vi "Main HMI.vi"() -> ()   [LabVIEW 2020]
uses:
  Control/State - Main HMI.ctl
  Control/Button Strip.ctl
  Control/State - eFGV.ctl
panel:
  in  "EXIT Button":bool
  out "error out":errorcluster
  in  "error in (no error)":errorcluster
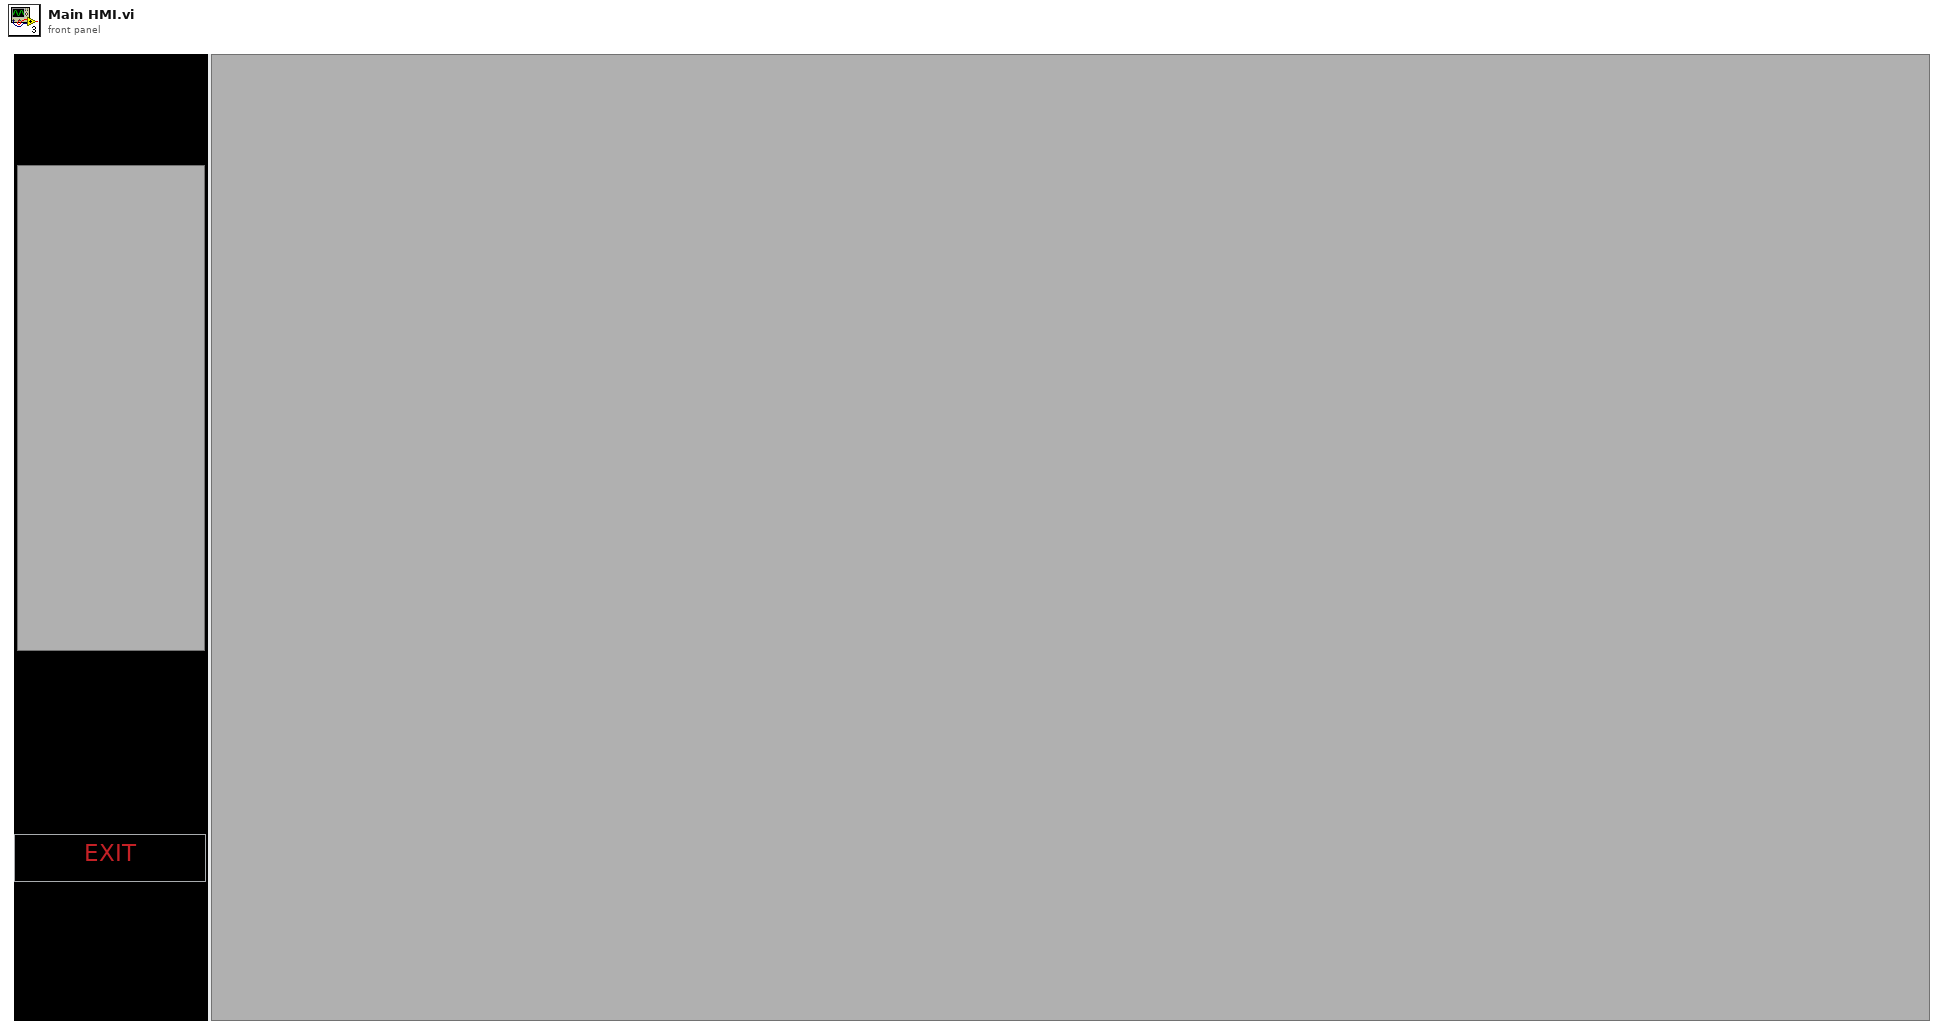
[diagram p1: front panel]
types:
  T1 = typedef "Button Strip.ctl" = enum32{"Home", "Setting", "Alert", "Save", "Chart"}
  T2 = cluster{"Timeout":i32, "Radio Buttons":T1, "All Module Ref":refnum<vi>[]}
  T3 = typedef "State - Main HMI.ctl" = enum16{"Init module", "Register event", "Init eFGV", "Run Module", "Idle", "Change Page", "Request Data from Modbus", "Process Data", "Update Layout", "Send to SQL Module", "Close All Module", "Unregister event", "Close module"}
  T4 = typedef "State - eFGV.ctl" = enum16{"Init", "Read", "Write", "Close"}
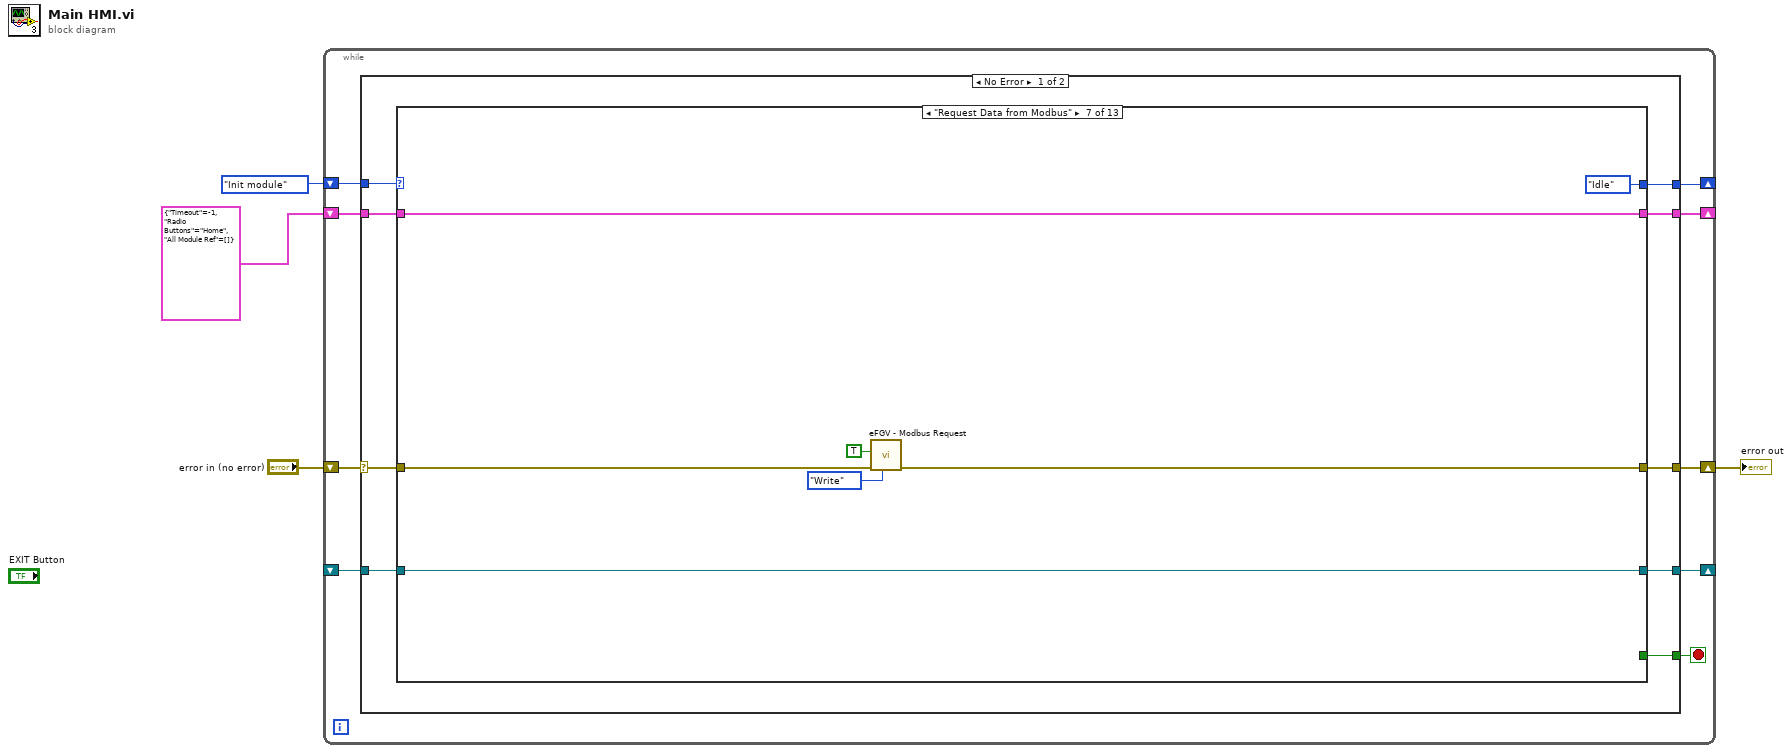
[diagram p0: block diagram]
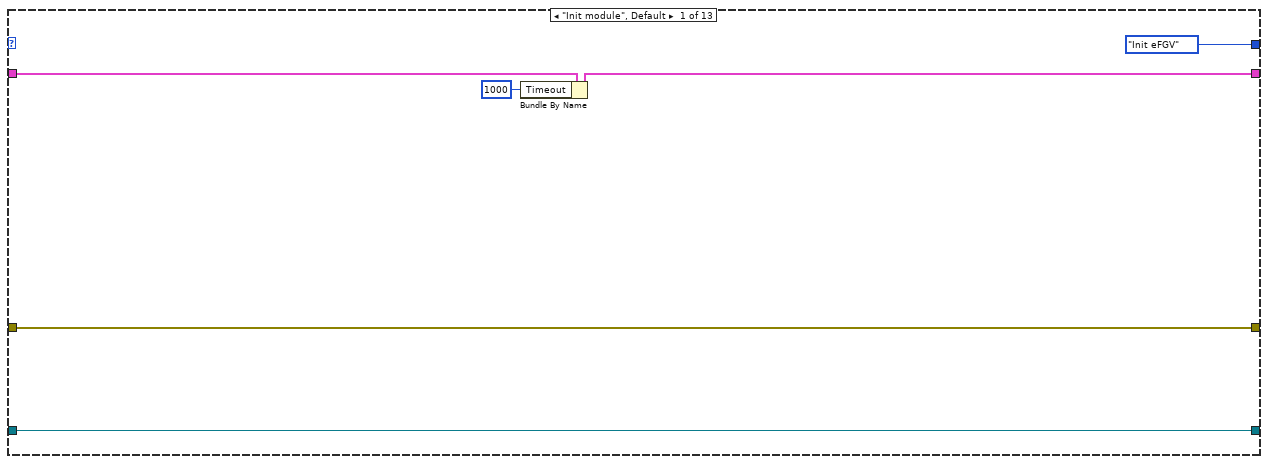
[diagram p2: hidden frame]
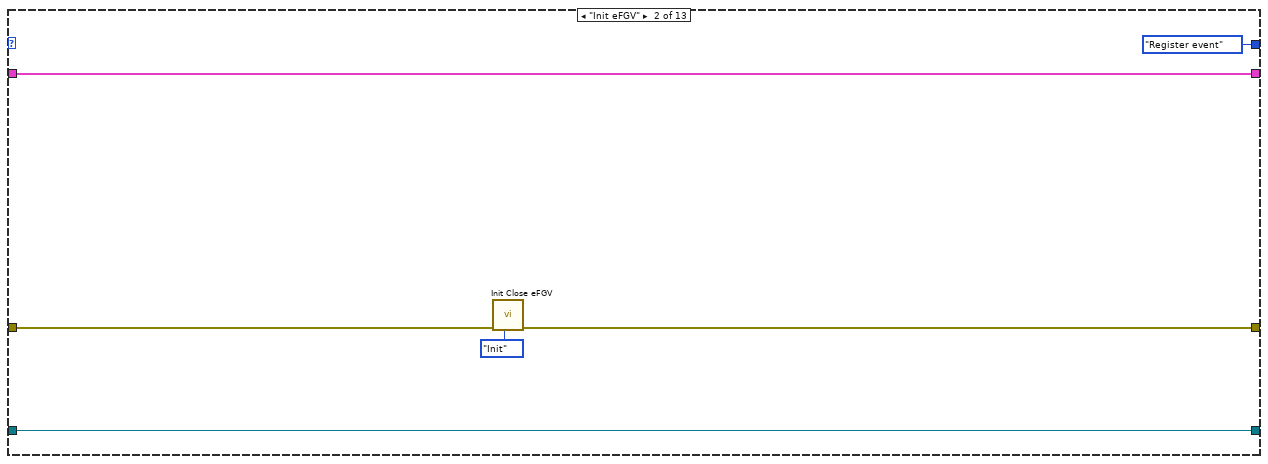
[diagram p3: hidden frame]
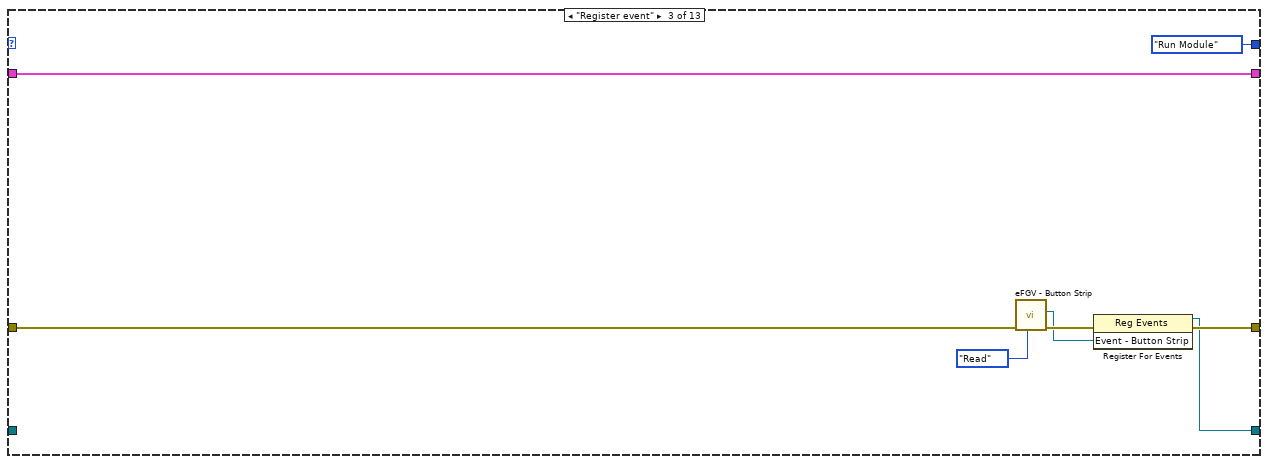
[diagram p4: hidden frame]
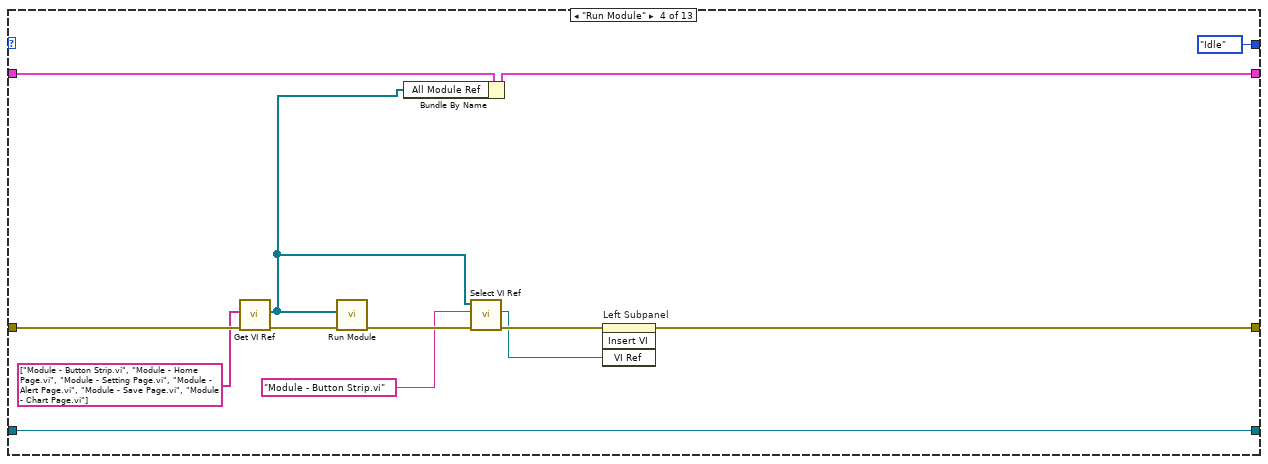
[diagram p5: hidden frame]
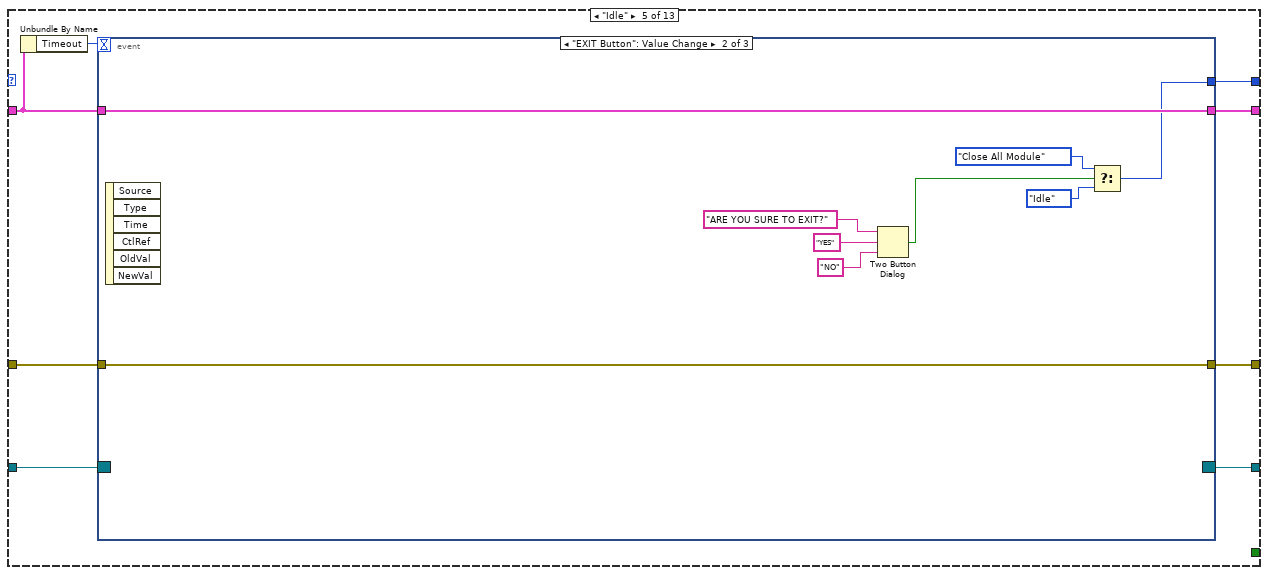
[diagram p6: hidden frame]
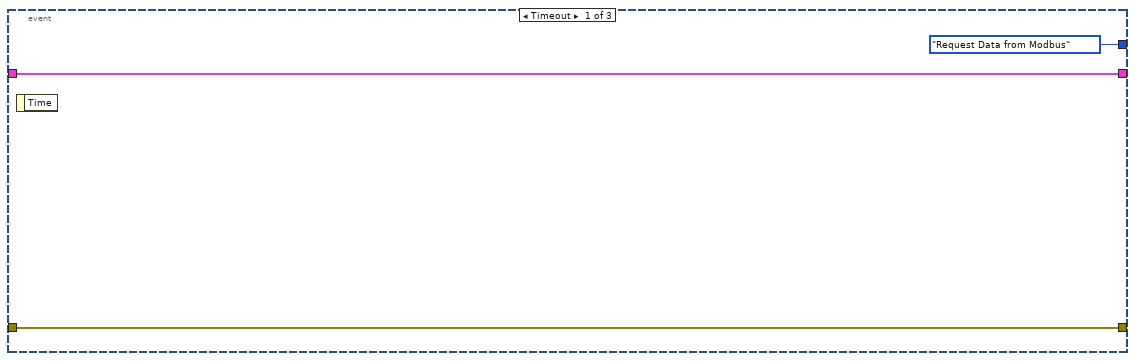
[diagram p7: hidden frame]
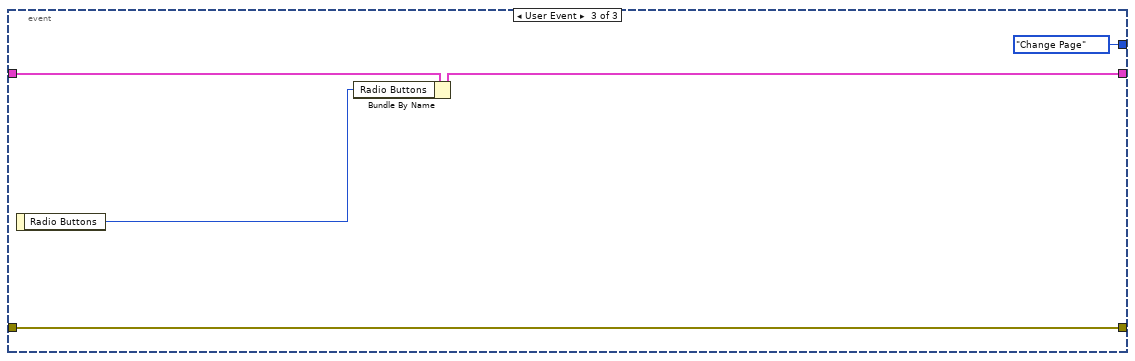
[diagram p8: hidden frame]
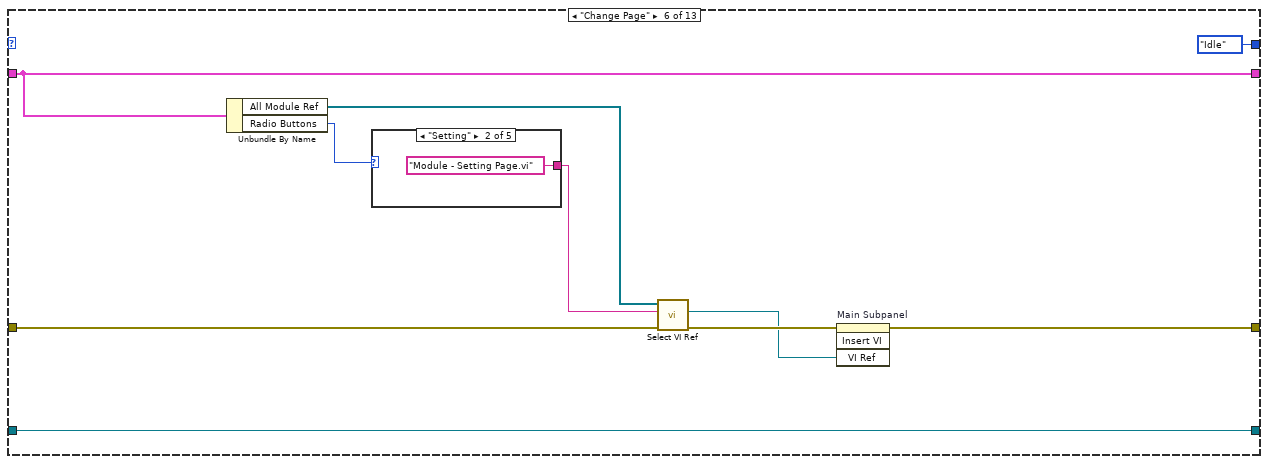
[diagram p9: hidden frame]
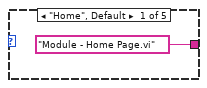
[diagram p10: hidden frame]
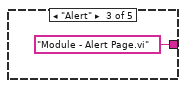
[diagram p11: hidden frame]
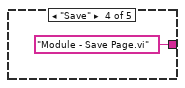
[diagram p12: hidden frame]
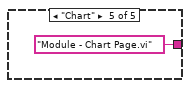
[diagram p13: hidden frame]
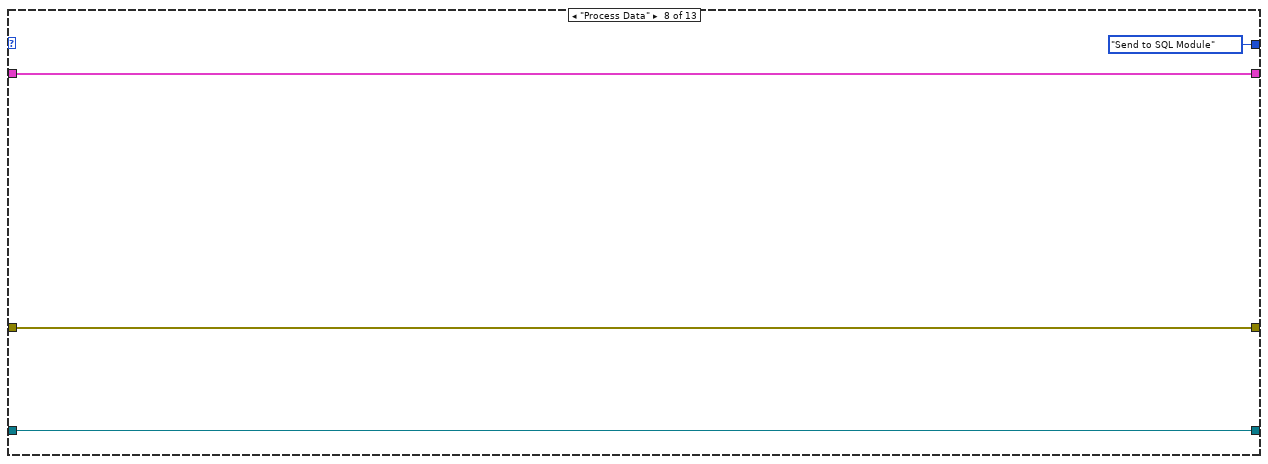
[diagram p14: hidden frame]
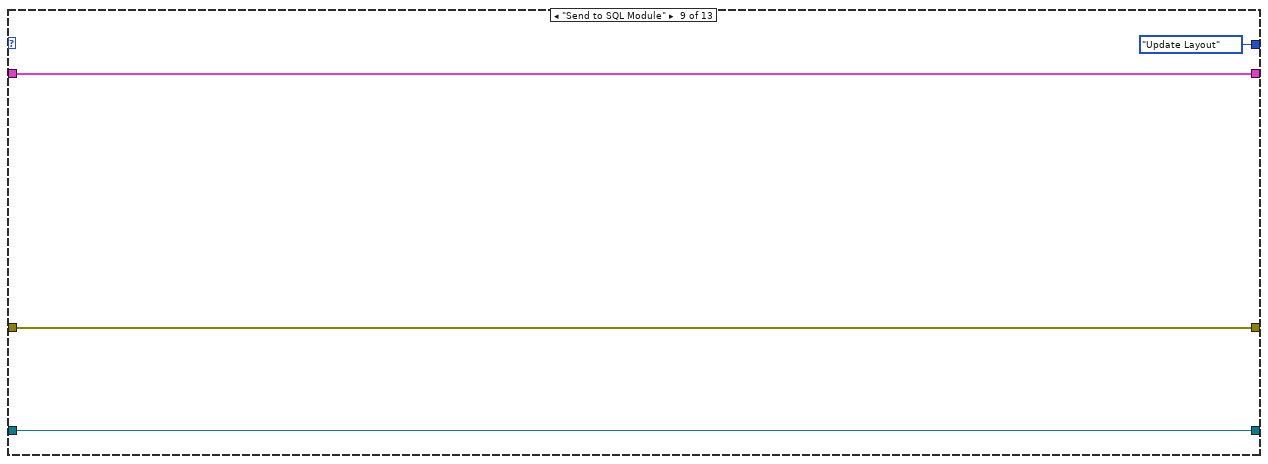
[diagram p15: hidden frame]
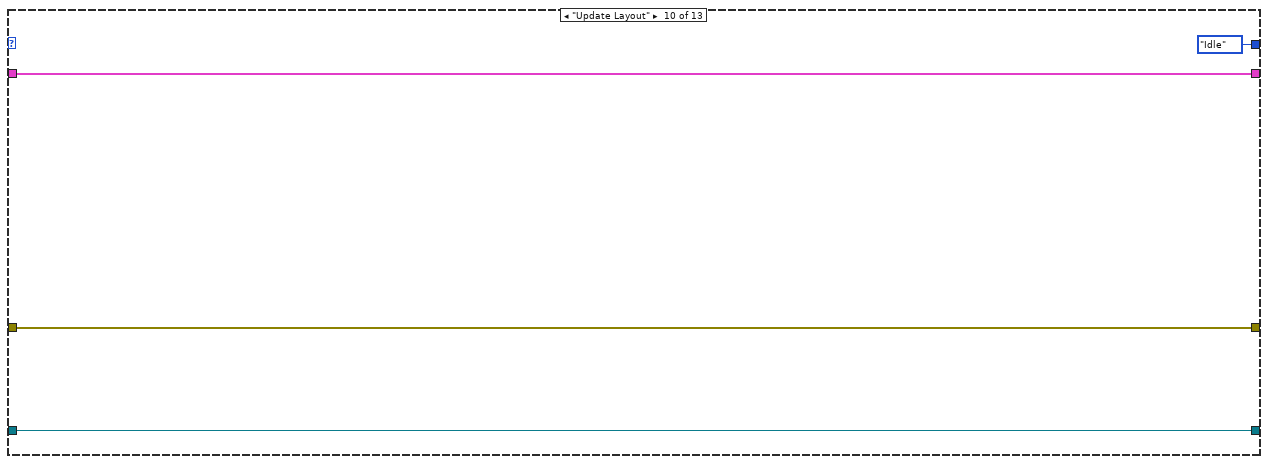
[diagram p16: hidden frame]
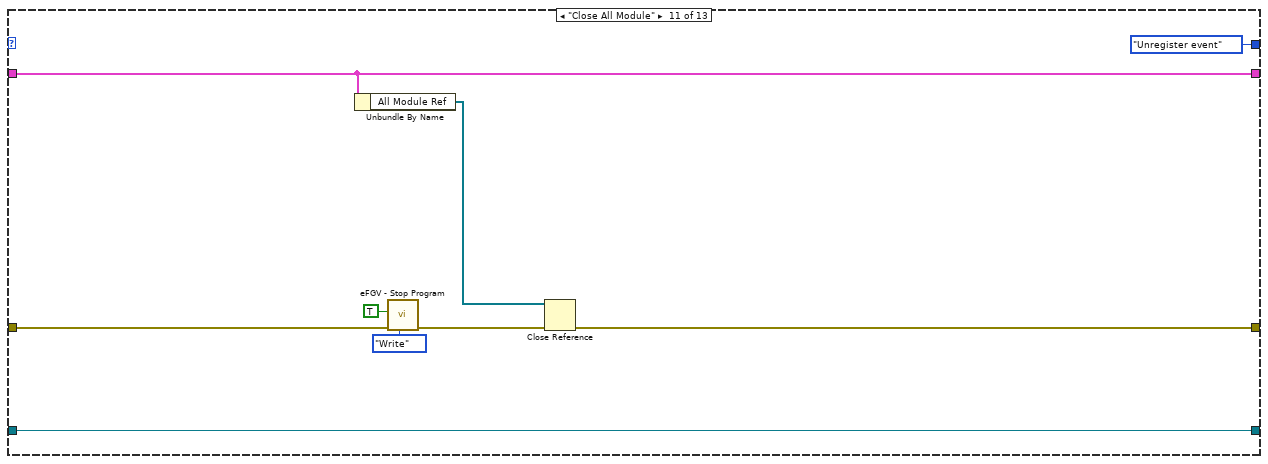
[diagram p17: hidden frame]
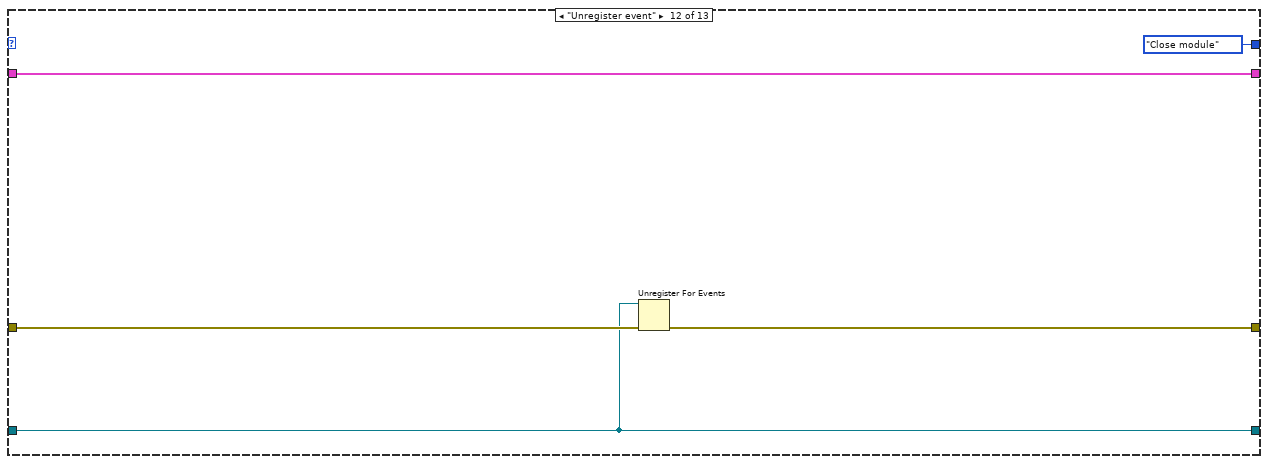
[diagram p18: hidden frame]
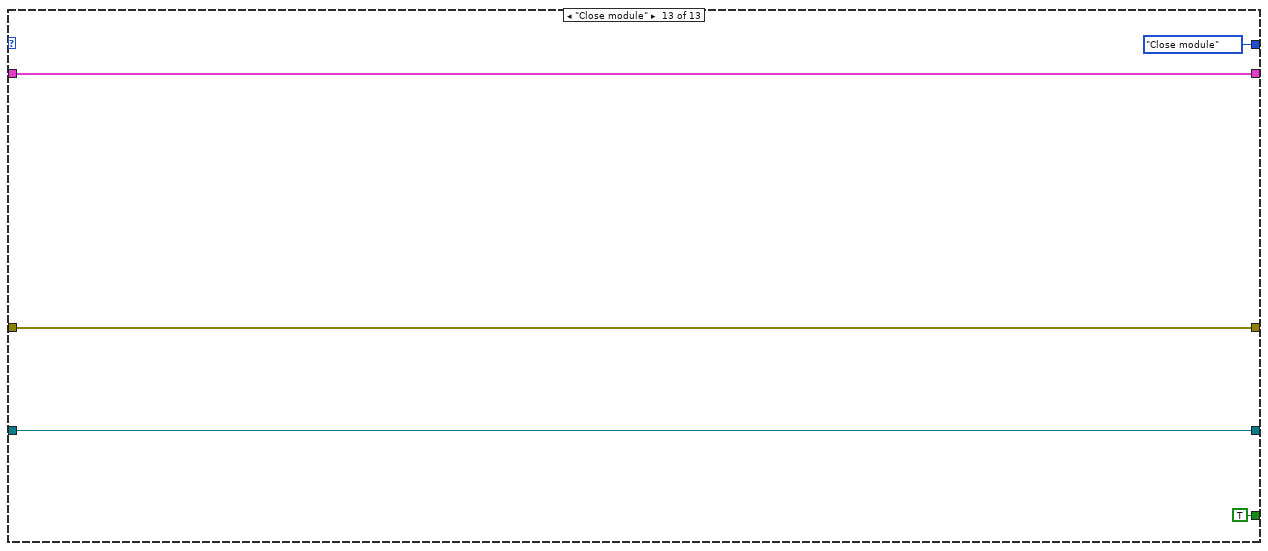
[diagram p19: hidden frame]
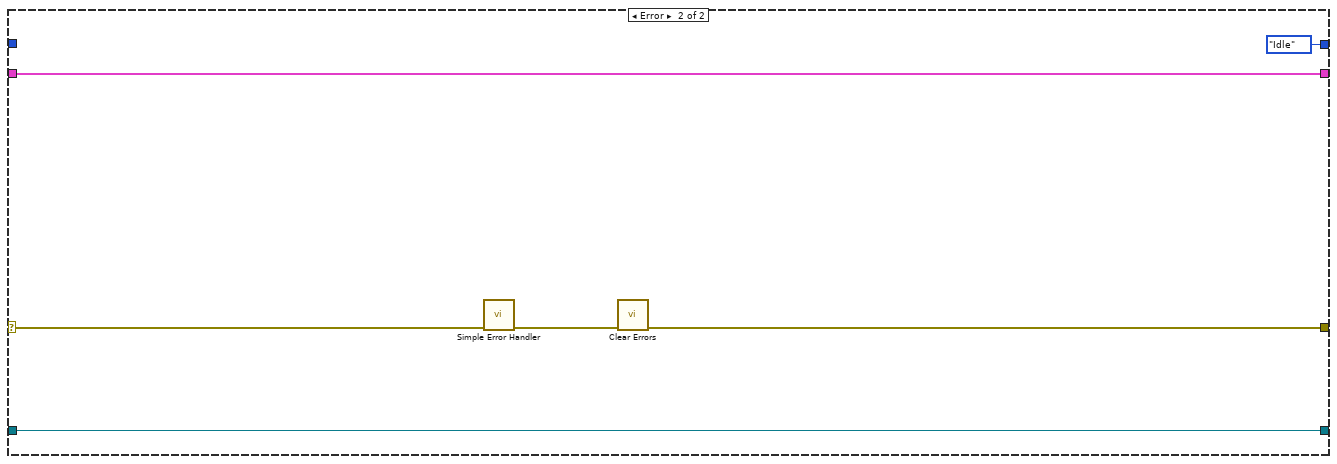
[diagram p20: hidden frame]
diagram:
  n1 = while {
    shift-right: [w11] -> w3
    shift-left: "error in (no error)" -> [w13]
    shift-right: [w7] -> _
    shift-left: State_-_Main_HMI."Init module" -> [w12]
    shift-right: [w9] -> _
    shift-left: T2 {"Timeout"=-1, "Radio Buttons"=enum."Home", "All Module Ref"=[]} -> [w10]
    shift-right: [w6] -> _
    shift-left: _ -> [w5]
    stop <- w8 stop-if-true
    n2 = case shown="No Error" w13 {
      selector: w13 -> [w21 w139]
      tunnel: w12 -> [w22 _]
      tunnel: [w20 w135] -> w11
      tunnel: w10 -> [w19 w137]
      tunnel: [w18 w137] -> w9
      tunnel: [w17 _] -> w8
      tunnel: [w16 State_-_Main_HMI."Idle"] -> w7
      tunnel: [w15 w134] -> w6
      tunnel: w5 -> [w14 w134]
      frame No Error {
        n3 = case shown="\"Request Data from Modbus\"" w22 {
          tunnel: w21 -> [w28 w31 w37 w54 w60 w87 w99 w106 w110 w114 w122 w127 w133]
          tunnel: [w28 w30 w40 w44 w59 w90 w98 w106 w110 w114 w116 w126 w133] -> w20
          tunnel: w19 -> [w27 w34 w42 w51 w62 w84 w102 w105 w109 w113 w118 w128 w132]
          tunnel: [w25 w34 w42 w50 w61 w84 w102 w105 w109 w113 w118 w128 w132] -> w18
          tunnel: [_ _ _ _ _ _ _ _ _ _ _ _ TRUE] -> w17
          tunnel: [State_-_Main_HMI."Init eFGV" State_-_Main_HMI."Register event" State_-_Main_HMI."Run Module" State_-_Main_HMI."Idle" w58 State_-_Main_HMI."Idle" State_-_Main_HMI."Idle" State_-_Main_HMI."Send to SQL Module" State_-_Main_HMI."Update Layout" State_-_Main_HMI."Idle" State_-_Main_HMI."Unregister event" State_-_Main_HMI."Close module" State_-_Main_HMI."Close module"] -> w16
          tunnel: [w23 w32 w39 w52 w56 w89 w100 w103 w107 w111 w119 w124 w129] -> w15
          tunnel: w14 -> [w23 w32 _ w52 w57 w89 w100 w103 w107 w111 w119 w124 w129]
          frame "Init module", Default {
            n4 = Bundle By Name(cluster=w27, "Timeout"=1000) -> (w25:T2)
          }
          frame "Init eFGV" {
            n5 = call "Init Close eFGV.vi"("State - eFGV"=State_-_eFGV."Init", "error in (no error)"=w31) -> ("error out"=w30:errorcluster)  [unwired: 9 in]
          }
          frame "Register event" {
            n6 = call "eFGV - Button Strip.vi"("State - eFGV"=State_-_eFGV."Read", "error in (no error)"=w37) -> ("error out"=w38:errorcluster, "Event - Button Strip"=w36:refnum<user-event>)  [unwired: 8 in]
            n7 = register-events(error in=w38, w36) -> (reference out=w39:refnum<event-registration>, error out=w40:errorcluster)  [unwired: 1 in]
          }
          frame "Run Module" {
            n8 = call "Get VI Ref.vi"("error in (no error)"=w54, "Module Names"=string[] ["Module - Button Strip.vi", "Module - Home Page.vi", "Module - Setting Page.vi", "Module - Alert Page.vi", "Module - Save Page.vi", "Module - Chart Page.vi"]) -> ("error out"=w49:errorcluster, "All Module Ref"=w47:refnum<vi>[])  [unwired: 8 in]
            n9 = call "Run Module.vi"("error in (no error)"=w49, "All Module Ref"=w47) -> ("error out"=w48:errorcluster)  [unwired: 9 in]
            n10 = Bundle By Name(cluster=w51, "All Module Ref"=w47) -> (w50:T2)
            n11 = call "Select VI Ref.vi"("error in (no error)"=w48, "Module Name"="Module - Button Strip.vi", "All Module Ref"=w47) -> ("error out"=w45:errorcluster, "VI Refnum"=w43:refnum<vi>)  [unwired: 7 in]
            n12 = invoke on="Left Subpanel" class="SubPnl" method="Insert VI"(error in=w45, "VI Ref"=w43) -> (error out=w44:errorcluster)  [unwired: 2 in, 3 out]
          }
          frame "Idle" {
            n13 = Unbundle By Name(w62) -> ("Timeout"=w63:i32)
            n14 = event shown="[1] \"EXIT Button\": Value Change" {
              selector: w57 -> [_ _ _]
              dyn-events: [_ _ _] -> w56
              timeout: w63 -> [_ _ _]
              tunnel: w62 -> [w66 w71 w80]
              tunnel: [w66 w71 w77] -> w61
              tunnel: w60 -> [w65 w72 w78]
              tunnel: [w65 w72 w78] -> w59
              tunnel: [State_-_Main_HMI."Request Data from Modbus" w68 State_-_Main_HMI."Change Page"] -> w58
              event Timeout {
                n15 = event-data() -> ()  [unwired: 1 in, 1 out]
              }
              event "EXIT Button": Value Change {
                n16 = event-data() -> ()  [unwired: 1 in, 6 out]
                n17 = Two Button Dialog(message="ARE YOU SURE TO EXIT?", 1:"NO" ("F button name (\"Cancel\")"), 2:"YES" ("T button name (\"OK\")")) -> (T button?=w67:bool)
                n18 = Select(t=State_-_Main_HMI."Close All Module", s=w67, f=State_-_Main_HMI."Idle") -> (s? t:f=w68:T3)
              }
              event User Event {
                n19 = event-data() -> ("Radio Buttons"=w76:T1)  [unwired: 1 in]
                n20 = Bundle By Name(cluster=w80, "Radio Buttons"=w76) -> (w77:T2)
              }
            }
          }
          frame "Change Page" {
            n21 = Unbundle By Name(w84) -> ("All Module Ref"=w83:refnum<vi>[], "Radio Buttons"=w82:T1)
            n22 = case shown="\"Setting\"" w82 {
              tunnel: ["Module - Home Page.vi" "Module - Setting Page.vi" "Module - Alert Page.vi" "Module - Save Page.vi" "Module - Chart Page.vi"] -> w81
              frame "Home", Default {
              }
              frame "Setting" {
              }
              frame "Alert" {
              }
              frame "Save" {
              }
              frame "Chart" {
              }
            }
            n23 = call "Select VI Ref.vi"("error in (no error)"=w87, "Module Name"=w81, "All Module Ref"=w83) -> ("error out"=w86:errorcluster, "VI Refnum"=w85:refnum<vi>)  [unwired: 7 in]
            n24 = invoke on="Main Subpanel" class="SubPnl" method="Insert VI"(error in=w86, "VI Ref"=w85) -> (error out=w90:errorcluster)  [unwired: 2 in, 3 out]
          }
          frame "Request Data from Modbus" {
            n25 = call "eFGV - Modbus Request.vi"("State - eFGV"=State_-_eFGV."Write", "error in (no error)"=w99, "Modbus Request"=TRUE) -> ("error out"=w98:errorcluster)  [unwired: 7 in, 1 out]
          }
          frame "Process Data" {
          }
          frame "Send to SQL Module" {
          }
          frame "Update Layout" {
          }
          frame "Close All Module" {
            n26 = Unbundle By Name(w118) -> ("All Module Ref"=w115:refnum<vi>[])
            n27 = call "eFGV - Stop Program.vi"("State - eFGV"=State_-_eFGV."Write", "error in (no error)"=w122, "Stop Program"=TRUE) -> ("error out"=w117:errorcluster)  [unwired: 7 in, 1 out]
            n28 = Close Reference(reference=w115, error in (no error)=w117) -> (error out=w116:errorcluster)
          }
          frame "Unregister event" {
            n29 = Unregister For Events(event registration refnum=w124, error in=w127) -> (error out=w126:errorcluster)
          }
          frame "Close module" {
          }
        }
      }
      frame Error {
        n30 = call <vilib>:"Simple Error Handler.vi"("error in (no error)"=w139) -> ("error out"=w138:errorcluster)  [unwired: 4 in, 4 out]
        n31 = call <vilib>:"Clear Errors.vi"("error in (no error)"=w138) -> ("error out"=w135:errorcluster)  [unwired: 5 in, 1 out]
      }
    }
  }
  "error out" <- w3
